vi "Recursive Combat.vi"(10 "Player 2 Deck":i32[](array[numeric]), 11 "Player 1 Deck":i32[](array[numeric])) -> (2 "Score":i32=33694, 3 "Player 1 wins":bool)   [LabVIEW 2020]
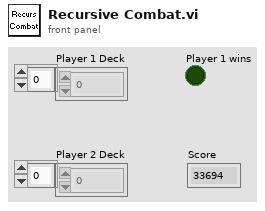
[diagram p1: front panel]
types:
  T1 = cluster{"Player 1 Deck":i32[], "Player 1 Deck 2":i32[]}
  T2 = set{cluster{"Player 1 Deck":i32[], "Player 1 Deck 2":i32[]}}
  T3 = cluster{"Player 1 Deck":i32[], "Player 2 Deck":i32[]}
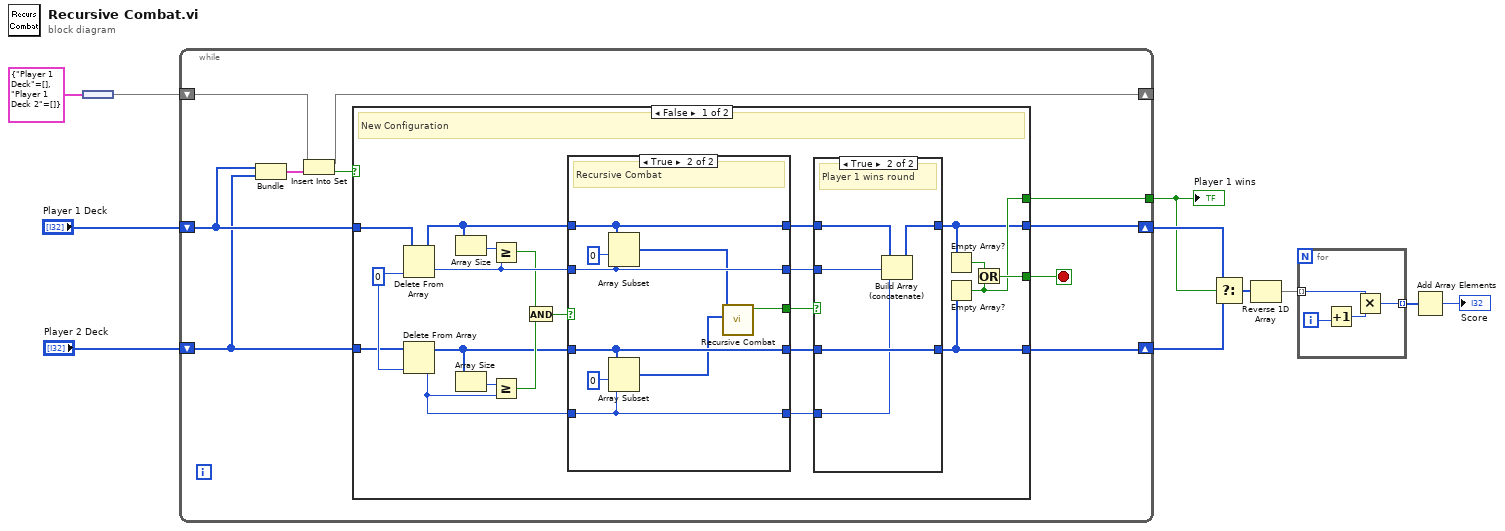
[diagram p0: block diagram]
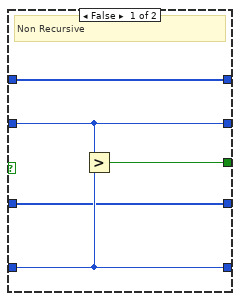
[diagram p2: hidden frame]
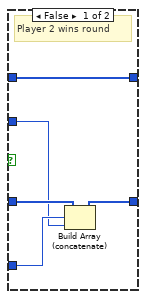
[diagram p3: hidden frame]
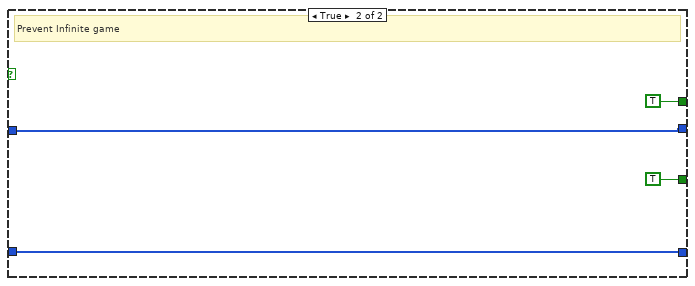
[diagram p4: hidden frame]
diagram:
  n1 = node(T1 {"Player 1 Deck"=[], "Player 1 Deck 2"=[]}) -> (w1:T2)
  n2 = while {
    shift-right: [w20] -> w10
    shift-left: "Player 1 Deck" -> [w17]
    shift-right: [w19] -> w11
    shift-left: "Player 2 Deck" -> [w16]
    shift-right: [w14] -> _
    shift-left: w1 -> [w18]
    tunnel: [w12] -> w3
    stop <- w21 stop-if-true
    n3 = Bundle("Player 1 Deck"=w17, "Player 2 Deck"=w16) -> (w15:T3)  [unwired: 1 in]
    n4 = Insert Into Set(10:w15, 11:w18) -> (2:w13:bool, 3:w14:T2)
    n5 = case shown="False" w13 {
      tunnel: [w43 TRUE] -> w21
      tunnel: [w36 w71] -> w20
      tunnel: [w35 w68] -> w19
      tunnel: w17 -> [w39 w71]
      tunnel: w16 -> [w38 w68]
      tunnel: [w37 TRUE ("empty?")] -> w12
      frame False {
        w41 = 0
        # "New Configuration"
        n6 = Delete From Array(array=w39, index=w41) -> (deleted portion=w33:i32, array with subset deleted=w27:i32[])  [unwired: 1 in]
        n7 = Delete From Array(array=w38, index=w41) -> (deleted portion=w31:i32, array with subset deleted=w26:i32[])  [unwired: 1 in]
        n8 = Array Size(array=w27) -> (size(s)=w34:i32)
        n9 = Array Size(array=w26) -> (size(s)=w32:i32)
        n10 = Greater Or Equal?(x=w34, y=w33) -> (x >= y?=w30:bool)
        n11 = Greater Or Equal?(x=w32, y=w31) -> (x >= y?=w29:bool)
        n12 = And(x=w30, y=w29) -> (x .and. y?=w28:bool)
        n13 = case shown="True" w28 {
          tunnel: [w48 w57] -> w40
          tunnel: w33 -> [w47 w55]
          tunnel: w31 -> [w46 w51]
          tunnel: w27 -> [w45 w56]
          tunnel: w26 -> [w44 w50]
          tunnel: [w45 w56] -> w25
          tunnel: [w44 w50] -> w24
          tunnel: [w47 w55] -> w23
          tunnel: [w46 w51] -> w22
          frame False {
            # "Non Recursive"
            n14 = Greater?(x=w47, y=w46) -> (0:w48:bool)
          }
          frame True {
            # "Recursive Combat"
            n15 = Array Subset(array=w56, index=0, length=w55) -> (w53:i32[])
            n16 = Array Subset(array=w50, index=0, length=w51) -> (w49:i32[])
            n17 = call "Recursive Combat.vi"("Player 2 Deck"=w49, "Player 1 Deck"=w53) -> ("Player 1 wins"=w57:bool)  [unwired: 8 in, 1 out]
          }
        }
        n18 = case shown="True" w40 {
          tunnel: w25 -> [w62 w64]
          tunnel: [w62 w63] -> w36
          tunnel: [w58 w67] -> w35
          tunnel: w24 -> [w61 w67]
          tunnel: w23 -> [w59 w66]
          tunnel: w22 -> [w60 w65]
          frame False {
            # "Player 2 wins round"
            n19 = Build Array (concatenate)(w61, w60, w59) -> (w58:i32[])
          }
          frame True {
            # "Player 1 wins round"
            n20 = Build Array (concatenate)(w64, w66, w65) -> (w63:i32[])
          }
        }
        n21 = Empty Array?(array=w36) -> (empty?=w42:bool)
        n22 = Empty Array?(array=w35) -> (empty?=w37:bool)
        n23 = Or(x=w42, y=w37) -> (x .or. y?=w43:bool)
      }
      frame True {
        # "Prevent Infinite game"
      }
    }
  }
  "Player 1 wins" <- w3
  n24 = Select(t=w10, s=w3, f=w11) -> (s? t:f=w6:i32[])
  n25 = Reverse 1D Array(array=w6) -> (reversed array=w7:i32[])
  n26 = for {
    tunnel: w7 -> [w73] mode=indexing
    tunnel: [w72] -> w8 mode=indexing
    i -> [w75]
    n27 = Increment(x=w75) -> (x+1=w74:i32)
    n28 = Multiply(x=w73, y=w74) -> (x*y=w72:i32)
  }
  n29 = Add Array Elements(numeric array=w8) -> (sum=→"Score":i32)
